vi "DAQ.Global.vi"() -> ()   [LabVIEW 2017, in "DAQ.lvlib"]
uses:
  DAQ.lvlib
panel:
  out "Safety":bool
  in  "Zamek2":bool
  in  "Zamek1":bool
  in  "Pull":bool
  in  "Push":bool
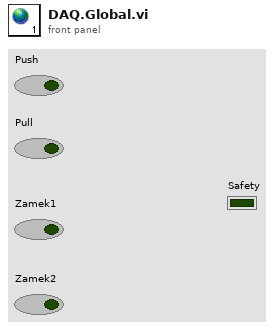
[diagram p1: front panel]
diagram:
